vi "State-Theta.vi"(0 "Slow Loop State in":T1 {"Phi Setpoint" format="%#_13g"}, 5 "IMU_sample_rate":i32=200, 9 "IMU Data Struct in":T3, 11 "error in":errorcluster) -> (10 "Fast Loop State out":T2, 15 "error out":errorcluster)   [LabVIEW 2014]
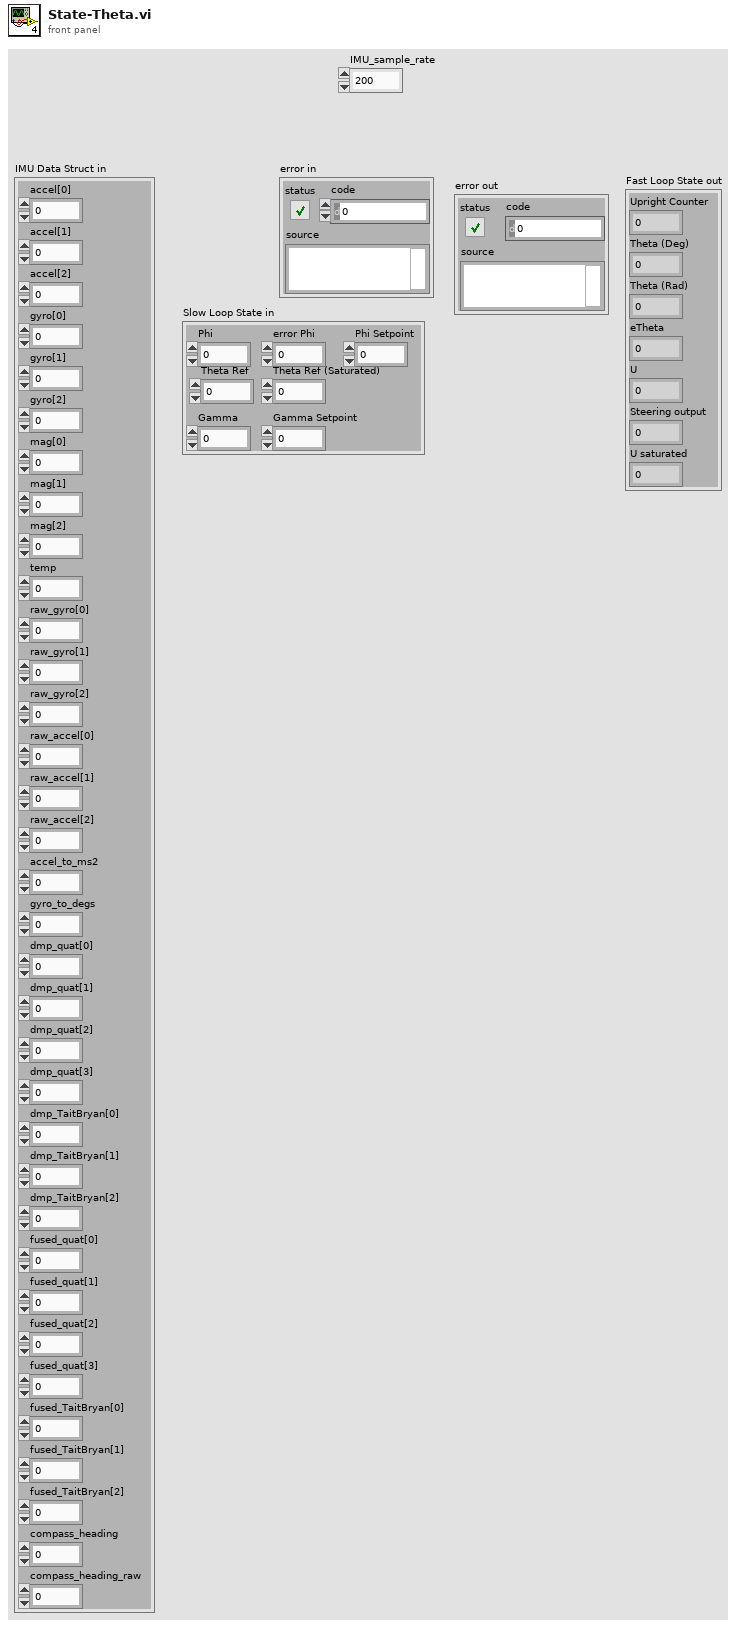
[diagram p1: front panel]
types:
  T1 = cluster{"Phi":dbl, "error Phi":dbl, "Gamma":dbl, "Theta Ref":dbl, "Theta Ref (Saturated)":sgl, "Gamma Setpoint":dbl, "Phi Setpoint":dbl}
  T2 = cluster{"Upright Counter":dbl, "Theta (Deg)":dbl, "Theta (Rad)":dbl, "eTheta":dbl, "U":dbl, "Steering output":dbl, "U saturated":sgl}
  T3 = cluster{"accel[0]":sgl, "accel[1]":sgl, "accel[2]":sgl, "gyro[0]":sgl, "gyro[1]":sgl, "gyro[2]":sgl, "mag[0]":sgl, "mag[1]":sgl, "mag[2]":sgl, "temp":sgl, "raw_gyro[0]":i16, "raw_gyro[1]":i16, "raw_gyro[2]":i16, "raw_accel[0]":i16, "raw_accel[1]":i16, "raw_accel[2]":i16, "accel_to_ms2":sgl, "gyro_to_degs":sgl, "dmp_quat[0]":sgl, "dmp_quat[1]":sgl, "dmp_quat[2]":sgl, "dmp_quat[3]":sgl, "dmp_TaitBryan[0]":sgl, "dmp_TaitBryan[1]":sgl, "dmp_TaitBryan[2]":sgl, "fused_quat[0]":sgl, "fused_quat[1]":sgl, "fused_quat[2]":sgl, "fused_quat[3]":sgl, "fused_TaitBryan[0]":sgl, "fused_TaitBryan[1]":sgl, "fused_TaitBryan[2]":sgl, "compass_heading":sgl, "compass_heading_raw":sgl}
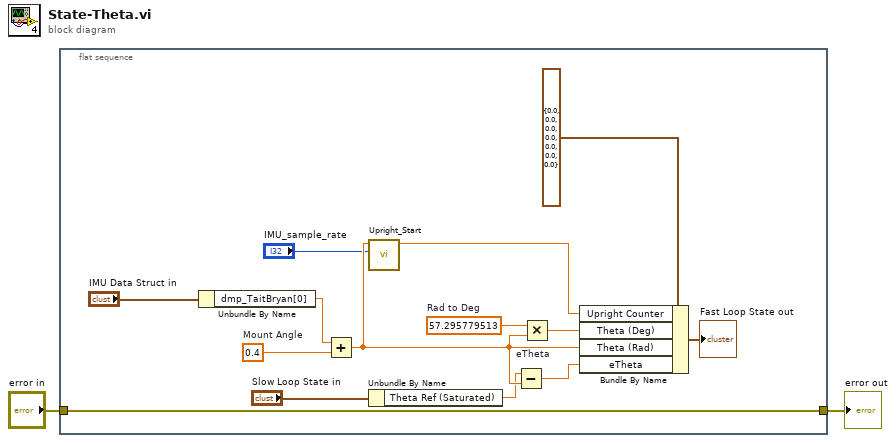
[diagram p0: block diagram]
diagram:
  n1 = flat-sequence {
    tunnel: "error in" -> [w12]
    tunnel: [w12] -> w1
    frame #0 {
      w15 = 0.4  # Mount Angle
      w14 = 57.295779513  # Rad to Deg
      n2 = Unbundle By Name("IMU Data Struct in") -> ("dmp_TaitBryan[0]"=w16:sgl)
      n3 = Add(x=w16, y=w15) -> (x+y=w7:dbl)
      n4 = call "Upright_Start.vi"("IMU_sample_rate"="IMU_sample_rate", "Current Theta"=w7) -> ("Upright Counter"=w9:dbl)  [unwired: 9 in]
      n5 = Unbundle By Name("Slow Loop State in") -> ("Theta Ref (Saturated)"=w5:sgl)
      n6 = Subtract "eTheta"(x=w5, y=w7) -> (x-y=w6:dbl)
      n7 = Multiply(x=w14, y=w7) -> (x*y=w8:dbl)
      n8 = Bundle By Name(cluster=T2 {"Upright Counter"=0.0, "Theta (Deg)"=0.0, "Theta (Rad)"=0.0, "eTheta"=0.0, "U"=0.0, "Steering output"=0.0, "U saturated"=0.0} ("State"), "Upright Counter"=w9, "Theta (Deg)"=w8, "Theta (Rad)"=w7, "eTheta"=w6) -> (→"Fast Loop State out":T2)
    }
  }
  "error out" <- w1
